vi "Get Service Class Instances.vi"() -> (3 "service instances":refnum<class "ServiceBase.lvclass">[](array[class]))   [LabVIEW 2021, in "CIFCorePlugin_server.lvlib"]
uses:
  CIFCorePlugin_server.lvlib
  <vilib>/gRPC/LabVIEW gRPC Servicer/ServiceBase/ServiceBase.lvclass
  RPC Service/PluginCore/PluginCore.lvclass
  C:/Program Files/National Instruments/LabVIEW 2021/vi.lib/gRPC/LabVIEW gRPC Servicer/ServiceBase/ServiceBase.lvclass
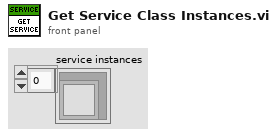
[diagram p1: front panel]
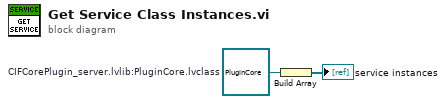
[diagram p0: block diagram]
diagram:
  w1 = refnum<class "PluginCore.lvclass"> refnum  # CIFCorePlugin_server.lvlib:PluginCore.lvclass
  n1 = Build Array(w1) -> (→"service instances":refnum<class "PluginCore.lvclass">[])
